vi "clLabview_updateFileReader.vi"(8 "clFileReader.lvclass OUT":refnum<class "clFileReader.lvclass">, 11 "vi_lib.lvlib:clLabview.lvclass":refnum<class "clLabview.lvclass">) -> (3 "vi_lib.lvlib:clLabview.lvclass 2":refnum<class "clLabview.lvclass">)   [LabVIEW 2020, in "vi_lib.lvlib" / "clLabview.lvclass"]
uses:
  clLabview.lvclass
  clFileReader/clFileReader.lvclass
  clLabview.lvclass/clLabview.ctl
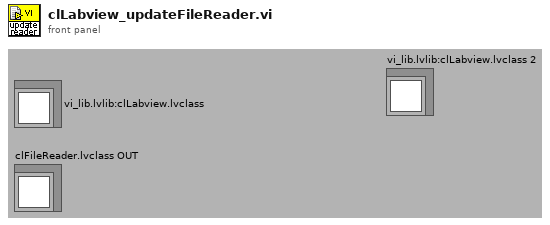
[diagram p1: front panel]
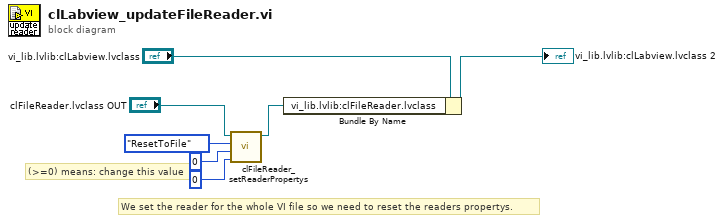
[diagram p0: block diagram]
diagram:
  # "(>=0) means: change this value"
  # "We set the reader for the whole VI file so we need to reset the readers propertys."
  n1 = call "clFileReader_setReaderPropertys.vi"("blocklen (>=0) if you want to change this value"=0 ("blocklen"), "hiddenoffset (>=0) if you want to change this value"=0 ("hiddenoffset"), "changeType"=enum16{"changeValues", "ResetToFile"}."ResetToFile", "clFileReader.lvclass IN"="clFileReader.lvclass OUT") -> ("clFileReader.lvclass OUT"=w4:refnum<class "clFileReader.lvclass">)  [unwired: 7 out]
  n2 = Bundle By Name(cluster="vi_lib.lvlib:clLabview.lvclass", "vi_lib.lvlib:clFileReader.lvclass"=w4) -> (→"vi_lib.lvlib:clLabview.lvclass 2":refnum<class "clLabview.lvclass">)
